vi "Init Lidar Labview.vi"(8 "error in (no error)":errorcluster) -> (0 "error out":errorcluster)   [LabVIEW 2017]
uses:
  <instrlib>/Hokuyo URG Series/Public/Initialize-Standard.vi
  Variables/Labview lidar globals.vi
  <instrlib>/Hokuyo URG Series/Hokuyo URG Series.lvlib
panel:
  out "return count":u32
  out "find list":string[](array[string])
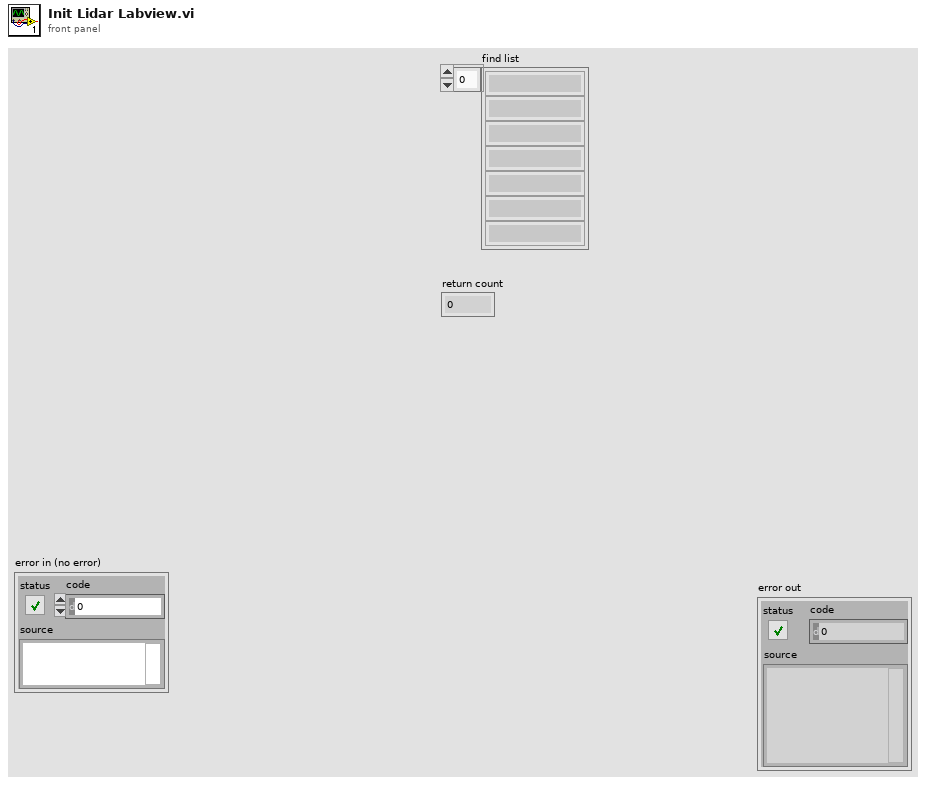
[diagram p1: front panel]
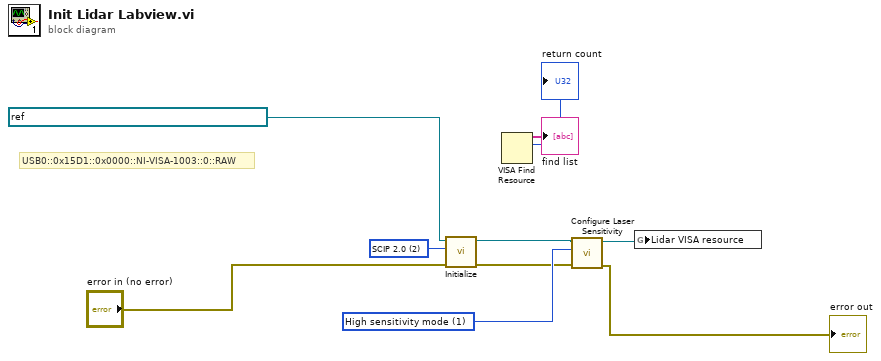
[diagram p0: block diagram]
diagram:
  w7 = u32 1 items=["Normal mode", "High sensitivity mode"] ("Sensitivity Mode (0: Normal mode)")
  w10 = u32 2 items=["Convert to Latest", "SCIP 1.1", "SCIP 2.0"] ("Protocol (2: SCIP 2.0)")
  # "USB0::0x15D1::0x0000::NI-VISA-1003::0::RAW"
  n1 = call-poly <instrlib>:"Initialize.vi"("error in (no error)"="error in (no error)", "Protocol (2: SCIP 2.0)"=w10, "VISA resource name"=refnum<visa-resource-name> "USB0::0x15D1::0x0000::NI-VISA-1003::1::RAW") -> ("error out"=w6:errorcluster, "VISA resource name out"=w8:refnum<visa-resource-name>)  [unwired: 7 in]
  n2 = VISA Find Resource() -> (2:→"return count":u32, 3:→"find list":string[])  [unwired: 3 in, 1 out]
  n3 = call <instrlib>:"Configure Laser Sensitivity.vi"("error in (no error)"=w6, "Sensitivity Mode (0: Normal mode)"=w7, "VISA resource name"=w8) -> ("error out"=→"error out":errorcluster, "VISA resource name out"=w4:refnum<visa-resource-name>)  [unwired: 7 in]
  n4 = global write "Labview lidar globals.vi" "Lidar VISA resource"(w4) -> ()
